vi "sub vi - Syringe Write.vi"(8 "error out":errorcluster, 10 "Command":string, 11 "VISA resource name out":refnum<visa-resource-name>) -> (0 "error out 2":errorcluster, 2 "Return String":string, 3 "VISA resource name out 2":refnum<visa-resource-name>)   [LabVIEW 2010]
panel:
  out "read buffer":string
  out "bytes read 4":u32
  in  "delay before read (ms) 4":u32=500
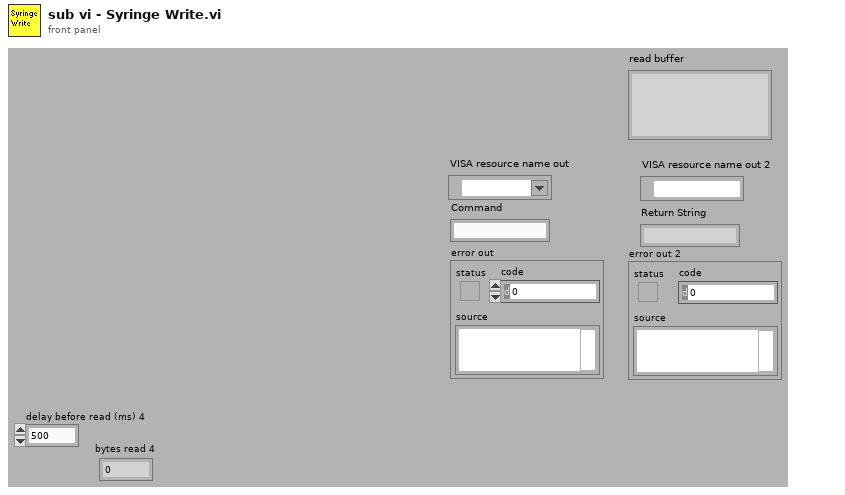
[diagram p1: front panel]
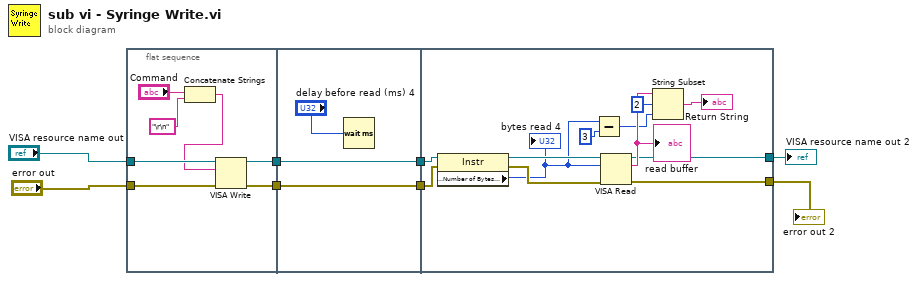
[diagram p0: block diagram]
diagram:
  n1 = flat-sequence {
    tunnel: "error out" -> [w15]
    tunnel: "VISA resource name out" -> [w14]
    tunnel: [w13] -> w8
    tunnel: [w12] -> w7
    tunnel: w8 -> [w18]
    tunnel: w7 -> [w17]
    tunnel: [w18] -> w6
    tunnel: [w17] -> w5
    tunnel: w6 -> [w26]
    tunnel: w5 -> [w28]
    tunnel: [w27] -> w1
    tunnel: [w20] -> w2
    frame #0 {
      n2 = Concatenate Strings("Command", "\r\n" ("string")) -> (w11:string)
      n3 = VISA Write(VISA resource name=w14, write buffer=w11, error in (no error)=w15) -> (VISA resource name out=w12:refnum<visa-resource-name>, error out=w13:errorcluster)  [unwired: 1 out]
    }
    frame #1 {
      n4 = Wait (ms)(milliseconds to wait="delay before read (ms) 4") -> ()  [unwired: 1 out]
    }
    frame #2 {
      n5 = property class="Instr"(reference=w28, error in=w26) -> (reference out=w30:refnum<visa-resource-name>, error out=w29:errorcluster, "Serial Settings:Number of Bytes at Serial Port"=w23:u32)
      "bytes read 4" <- w23
      n6 = Subtract(x=w23, y=u32 3) -> (x-y=w21:u32)
      n7 = VISA Read(VISA resource name=w30, byte count=w23, error in (no error)=w29) -> (VISA resource name out=w20:refnum<visa-resource-name>, read buffer=w25:string, error out=w27:errorcluster)  [unwired: 1 out]
      "read buffer" <- w25
      n8 = String Subset(string=w25, offset (0)=2, length (rest)=w21) -> (substring=→"Return String":string)
    }
  }
  "VISA resource name out 2" <- w2
  "error out 2" <- w1
